vi "ep_Simulate Basic Breaker.vi"(0 "trip pulse signal? (F)":bool, 5 "close pulse signal? (F)":bool, 9 "interrupting time [ms]":u32, 11 "closing time [ms]":u32) -> (4 "breaker closed?":bool)   [LabVIEW 2012]
uses:
  <vilib>/addons/Electrical Power/Protection/NI_EP_Protection_FPGA.lvlib
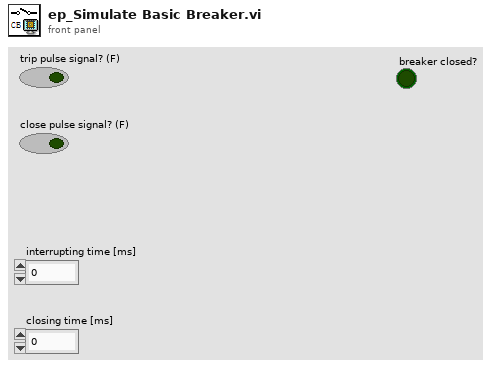
[diagram p1: front panel]
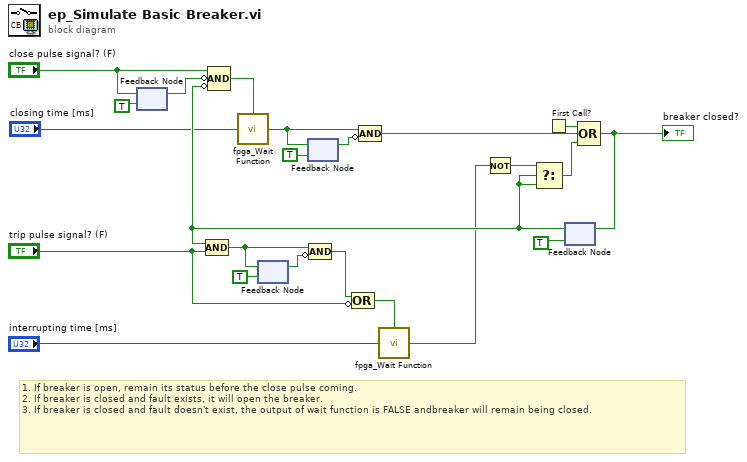
[diagram p0: block diagram]
diagram:
  # "1. If breaker is open, remain its status before the close pulse coming.\n2. If breaker is closed and fault exists, it will open the breaker.\n3. If breaker is closed and fault doesn't exist, the output of wait function is FALSE andbreaker will remain being closed."
  n1 = feedback #1(TRUE) -> (w15:bool)
  n2 = feedback-in #1("close pulse signal? (F)") -> ()
  n3 = feedback #2(TRUE) -> (w19:bool)
  n4 = feedback #3(TRUE) -> (w7:bool)
  n5 = First Call?() -> (First Call?: T/F=w22:bool)
  n6 = feedback #4(TRUE) -> (w10:bool)
  n7 = Compound Arithmetic op=AND(w10, "trip pulse signal? (F)") -> (w21:bool)
  n8 = Compound Arithmetic op=AND("close pulse signal? (F)", invert w15, invert w10) -> (w9:bool)
  n9 = call <vilib>:"fpga_Wait Function.vi"("start? (F)"=w9, "timeout (ms)"="closing time [ms]") -> ("timeout?"=w6:bool)  [unwired: 13 in]
  n10 = feedback-in #2(w21) -> ()
  n11 = feedback-in #3(w6) -> ()
  n12 = Compound Arithmetic op=AND(w21, invert w19) -> (w23:bool)
  n13 = Compound Arithmetic op=OR(w23, invert "trip pulse signal? (F)") -> (w12:bool)
  n14 = Compound Arithmetic op=AND(w6, invert w7) -> (w4:bool)
  n15 = call <vilib>:"fpga_Wait Function.vi"("start? (F)"=w12, "timeout (ms)"="interrupting time [ms]") -> ("timeout?"=w2:bool)  [unwired: 13 in]
  n16 = Not(x=w2) -> (.not. x?=w1:bool)
  n17 = Select(t=w1, s=w10, f=w10) -> (s? t:f=w18:bool)
  n18 = Compound Arithmetic op=OR(w22, w4, w18) -> (w17:bool)
  "breaker closed?" <- w17
  n19 = feedback-in #4(w17) -> ()
